vi "Write Results to VS Engine.vi"(8 "Error In":errorcluster, 10 "Results Data":dbl[](array[numeric]), 11 "VS Return Block Data Refs":T1 {"Block Data Refs"."Data Reference" format="%.0x"}) -> (0 "Error Out":errorcluster)   [LabVIEW 2014, in "Waveform-Processing-Custom-Device Engine.lvlib"]
uses:
  Waveform-Processing-Custom-Device Engine.lvlib
  Shared/VS Return Block Data Refs.ctl
  <vilib>/NI Veristand/Custom Device API/Block Data Reference.ctl
  <vilib>/NI Veristand/Custom Device API/Data Reference.ctl
  <vilib>/NI Veristand/Custom Device API/Custom Device API.lvlib
  Shared/Waveform-Processing-Custom-Device Shared.lvlib
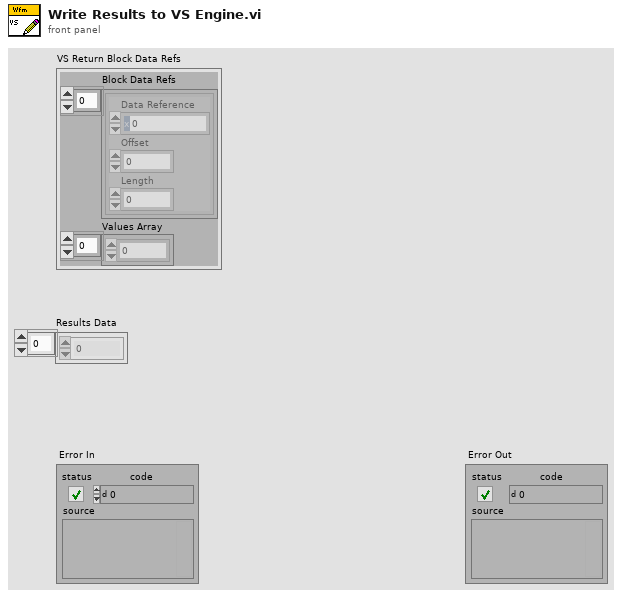
[diagram p1: front panel]
types:
  T1 = typedef "Waveform-Processing-Custom-Device Shared.lvlib/VS Return Block Data Refs.ctl" = cluster{"Block Data Refs":T2[], "Values Array":dbl[]}
  T2 = typedef "Custom Device API.lvlib/Block Data Reference.ctl" = cluster{"Data Reference":T3, "Offset":i32, "Length":i32}
  T3 = typedef "Custom Device API.lvlib/Data Reference.ctl" = i32
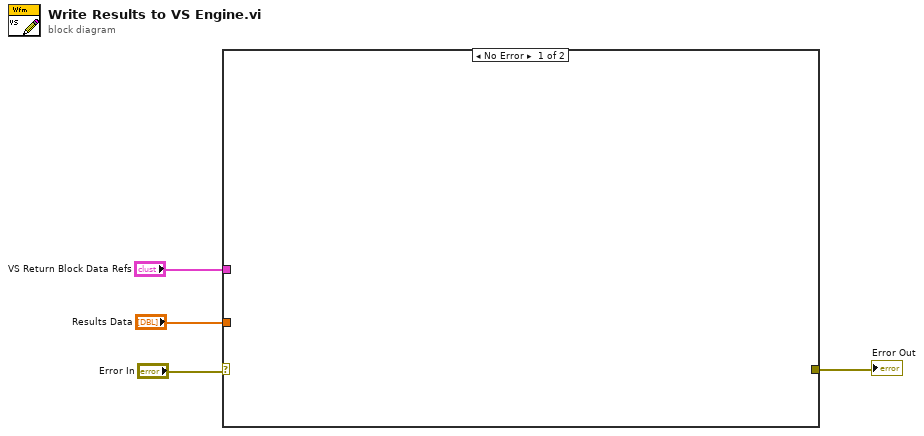
[diagram p0: block diagram]
diagram:
  n1 = case shown="No Error" "Error In" {
    selector: "Error In" -> [_ w5]
    tunnel: "Results Data" -> [_ _]
    tunnel: "VS Return Block Data Refs" -> [_ _]
    tunnel: [_ w5] -> w1
    frame No Error {
    }
    frame Error {
    }
  }
  "Error Out" <- w1
